vi "Robot Values.vi"() -> ()   [LabVIEW 2016]
uses:
  Robot Values.ctl
panel:
  in  "Robot Values":T1
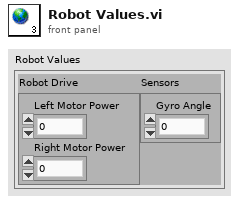
[diagram p1: front panel]
types:
  T1 = typedef "Robot Values.ctl" = cluster{"Robot Drive":cluster{"Left Motor Power":dbl, "Right Motor Power":dbl}, "Sensors":cluster{"Gyro Angle":dbl}}
diagram:
